vi "Test Class.vi"() -> ()   [LabVIEW 2020]
uses:
  Hardware/Actuators/Servos/Simulated Servo/Simulated Servo.lvclass
  C:/Users/jharw/Documents/1 Folder to Rule them All/UMD/Inflation-Apparatus/src/Hardware/Actuators/Servos/Servo.lvclass
  Hardware/Sensors/Cameras/Simulated Camera/Simulated Camera.lvclass
  C:/Users/jharw/Documents/1 Folder to Rule them All/UMD/Inflation-Apparatus/src/Hardware/Sensors/Cameras/Camera.lvclass
  Hardware/Sensors/Force Sensors/Simulated Force Sensor/Simulated Force Sensor.lvclass
  C:/Users/jharw/Documents/1 Folder to Rule them All/UMD/Inflation-Apparatus/src/Hardware/Sensors/Force Sensors/Force Sensor.lvclass
  Hardware/Actuators/Switches/Simulated Switch/Simulated Switch.lvclass
  C:/Users/jharw/Documents/1 Folder to Rule them All/UMD/Inflation-Apparatus/src/Hardware/Actuators/Switches/Switch.lvclass
  Hardware/Actuators/Switches/Switch.lvclass/Switch.ctl
  Hardware/Sensors/Force Sensors/Force Sensor.lvclass/Force Sensor.ctl
  Hardware/Sensors/Cameras/Camera.lvclass/Camera.ctl
  Hardware/Actuators/Servos/Servo.lvclass/Servo.ctl
  Hardware/Sensors/Force Sensors/Force Sensor.lvclass
  Hardware/Sensors/Cameras/Camera.lvclass
  Hardware/Actuators/Servos/Servo.lvclass
  Hardware/Actuators/Switches/Switch.lvclass
panel:
  in  "switch state":bool
  in  "pulse width (micro-sec)":dbl
  out "current image":T1(plugin-control)
  out "diameter (mm)":dbl
  out "force (V)":dbl
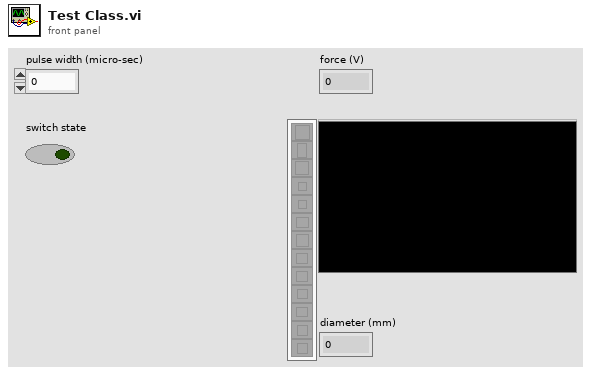
[diagram p1: front panel]
types:
  T1 = typedef "IMAQ Image.ctl" = refnum<image>
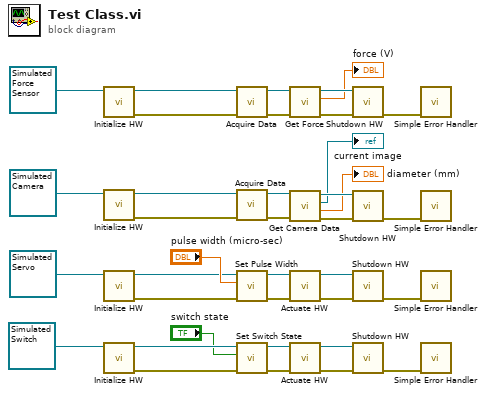
[diagram p0: block diagram]
diagram:
  n1 = call-dynamic "Initialize HW.vi"("Simulated Force Sensor in"=refnum<class "Simulated Force Sensor.lvclass"> refnum ("Simulated Force Sensor.lvclass")) -> ("error out"=w35:errorcluster, "Simulated Force Sensor out"=w36:refnum<class "Simulated Force Sensor.lvclass">)  [unwired: 9 in]
  n2 = call-dynamic "Initialize HW.vi"("Camera in"=refnum<class "Simulated Camera.lvclass"> refnum ("Simulated Camera.lvclass")) -> ("error out"=w28:errorcluster, "Camera out"=w26:refnum<class "Simulated Camera.lvclass">)  [unwired: 9 in]
  n3 = call-dynamic "Initialize HW.vi"("Simulated Servo in"=refnum<class "Simulated Servo.lvclass"> refnum ("Simulated Servo.lvclass")) -> ("error out"=w17:errorcluster, "Simulated Servo out"=w13:refnum<class "Simulated Servo.lvclass">)  [unwired: 9 in]
  n4 = call-dynamic "Initialize HW.vi"("Simulated Switch in"=refnum<class "Simulated Switch.lvclass"> refnum ("Simulated Switch.lvclass")) -> ("error out"=w2:errorcluster, "Simulated Switch out"=w8:refnum<class "Simulated Switch.lvclass">)  [unwired: 9 in]
  n5 = call-dynamic "Acquire Data.vi"("error in (no error)"=w35, "Simulated Force Sensor in"=w36) -> ("error out"=w33:errorcluster, "Simulated Force Sensor out"=w34:refnum<class "Simulated Force Sensor.lvclass">)  [unwired: 8 in]
  n6 = call-dynamic "Acquire Data.vi"("error in (no error)"=w28, "Simulated Camera in"=w26) -> ("error out"=w24:errorcluster, "Simulated Camera out"=w25:refnum<class "Simulated Camera.lvclass">)  [unwired: 8 in]
  n7 = call "Set Pulse Width.vi"("error in (no error)"=w17, "pulse width (micro-sec)"="pulse width (micro-sec)", "Servo in"=w13) -> ("error out"=w16:errorcluster, "Servo out"=w11:refnum<class "Simulated Servo.lvclass">)  [unwired: 7 in]
  n8 = call "Set Switch State.vi"("error in (no error)"=w2, "switch state"="switch state", "Switch in"=w8) -> ("error out"=w3:errorcluster, "Switch out"=w7:refnum<class "Simulated Switch.lvclass">)  [unwired: 7 in]
  n9 = call "Get Force.vi"("error in (no error)"=w33, "Force Sensor in"=w34) -> ("error out"=w32:errorcluster, "force (V)"=→"force (V)":dbl, "Force Sensor out"=w31:refnum<class "Simulated Force Sensor.lvclass">)  [unwired: 7 in]
  n10 = call "Get Camera Data.vi"("error in (no error)"=w24, "Camera in"=w25) -> ("error out"=w22:errorcluster, "diameter (mm)"=→"diameter (mm)":dbl, "image"=→"current image":T1, "Camera out"=w23:refnum<class "Simulated Camera.lvclass">)  [unwired: 6 in]
  n11 = call-dynamic "Actuate HW.vi"("error in (no error)"=w16, "Simulated Servo in"=w11) -> ("error out"=w15:errorcluster, "Simulated Servo out"=w10:refnum<class "Simulated Servo.lvclass">)  [unwired: 8 in]
  n12 = call-dynamic "Actuate HW.vi"("error in (no error)"=w3, "Simulated Switch in"=w7) -> ("error out"=w4:errorcluster, "Simulated Switch out"=w6:refnum<class "Simulated Switch.lvclass">)  [unwired: 8 in]
  n13 = call-dynamic "Shutdown HW.vi"("error in (no error)"=w32, "Simulated Force Sensor in"=w31) -> ("error out"=w29:errorcluster)  [unwired: 8 in, 1 out]
  n14 = call-dynamic "Shutdown HW.vi"("error in (no error)"=w22, "Camera in"=w23) -> ("error out"=w21:errorcluster)  [unwired: 8 in, 1 out]
  n15 = call-dynamic "Shutdown HW.vi"("error in (no error)"=w15, "Simulated Servo in"=w10) -> ("error out"=w14:errorcluster)  [unwired: 8 in, 1 out]
  n16 = call-dynamic "Shutdown HW.vi"("error in (no error)"=w4, "Simulated Switch in"=w6) -> ("error out"=w5:errorcluster)  [unwired: 8 in, 1 out]
  n17 = call <vilib>:"Simple Error Handler.vi"("error in (no error)"=w29) -> ()  [unwired: 4 in, 5 out]
  n18 = call <vilib>:"Simple Error Handler.vi"("error in (no error)"=w21) -> ()  [unwired: 4 in, 5 out]
  n19 = call <vilib>:"Simple Error Handler.vi"("error in (no error)"=w14) -> ()  [unwired: 4 in, 5 out]
  n20 = call <vilib>:"Simple Error Handler.vi"("error in (no error)"=w5) -> ()  [unwired: 4 in, 5 out]
